vi "Set Analog In Trigger Detector.vi"(0 "hdwf":i32, 1 "voltsLevel":dbl, 2 "HystersisvoltsLevel":dbl, 5 "idxChannel":i32, 7 "trigcond":T3, 9 "trigtype":T2, 11 "error in (no error)":errorcluster, 12 "filter":T1=enum."Average") -> (4 "hdwf out":i32, 15 "error out":errorcluster)   [LabVIEW 2014, in "AnalogDiscSDKLv.lvlib"]
doc: "extern \"C\" __declspec(dllexport) int Set_AnalogIn_TriggerDetector(HDWF hdwf, \n int idxChannel, TRIGCOND trigcond, TRIGTYPE trigtype, double voltsLevel, FILTER filter, double HystersisvoltsLEvel );"
uses:
  <instrlib>/AnalogDiscSDKLv/AnalogDiscSDKLv.lvlib
  <instrlib>/AnalogDiscSDKLv/VIs/DWF_TrigCond.ctl
  <instrlib>/AnalogDiscSDKLv/VIs/DWF_TrigType.ctl
  <instrlib>/AnalogDiscSDKLv/VIs/DWF_Filter.ctl
  <instrlib>/AnalogDiscSDKLv/AnalogDiscSDKLv.dll
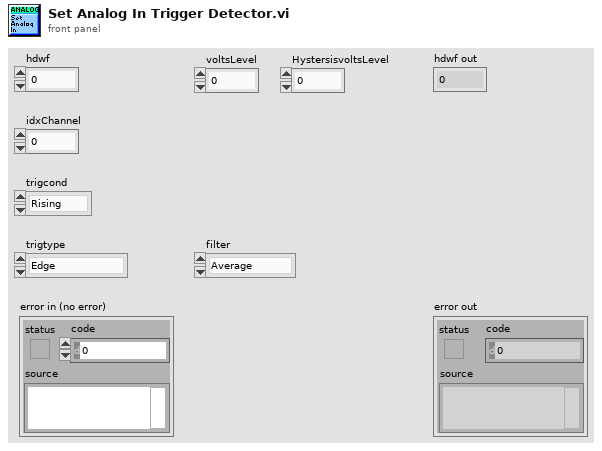
[diagram p1: front panel]
types:
  T1 = typedef "AnalogDiscSDKLv.lvlib/DWF_Filter.ctl" = enum16{"Decimate", "Average", "MinMax"}
  T2 = typedef "AnalogDiscSDKLv.lvlib/DWF_TrigType.ctl" = enum16{"Edge", "Pulse", "Transition"}
  T3 = typedef "AnalogDiscSDKLv.lvlib/DWF_TrigCond.ctl" = enum16{"Rising", "Falling"}
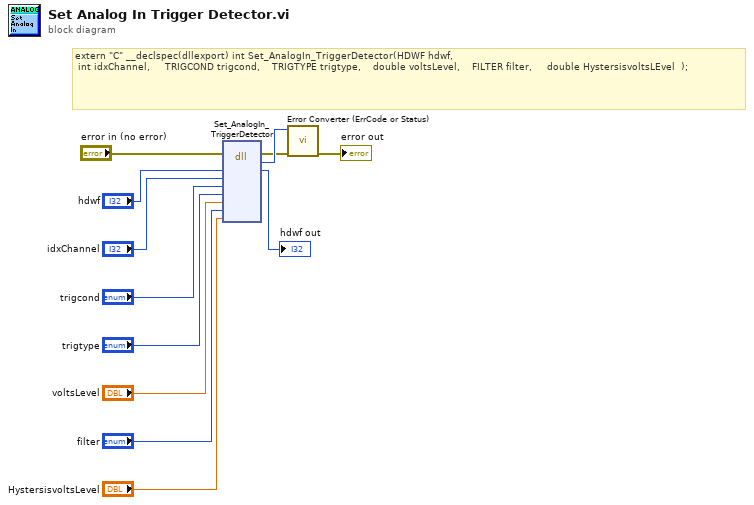
[diagram p0: block diagram]
diagram:
  # "extern \"C\" __declspec(dllexport) int Set_AnalogIn_TriggerDetector(HDWF hdwf, \n\tint idxChannel,\t\t\t\t\tTRIGCOND trigcond,\t\t\t\tTRIGTYPE trigtype,\t\t\t\tdouble voltsLevel,\t\t\t\tFILTER filter,\t\t\t\t\tdouble HystersisvoltsLEvel\t\t);"
  n1 = dll-call lib="C:/Program Files (x86)/National Instruments/LabVIEW 2014/instr.lib/AnalogDiscSDKLv/AnalogDiscSDKLv.*" fn="Set_AnalogIn_TriggerDetector"(error in="error in (no error)", "hdwf"="hdwf", "idxChannel"="idxChannel", "trigcond"="trigcond", "trigtype"="trigtype", "voltsLevel"="voltsLevel", "filter"="filter", "HystersisvoltsLEvel"="HystersisvoltsLevel") -> (error out=w2:errorcluster, w12:i32, "hdwf"=→"hdwf out":i32)  [unwired: 8 in, 1 out]
  n2 = call <instrlib>:"Error Converter (ErrCode or Status).vi"("error in (no error)"=w2, "error code"=w12) -> ("error out"=→"error out":errorcluster)  [unwired: 9 in]
